vi "U3 Firmware Counter with Debounce.vi"() -> ()   [LabVIEW 2021]
panel:
  in  "Rising Edges":bool
  in  "Debounce Period Values":u8[](array[numeric])=[50, 50]
  out "Counter Reads":u32[](array[numeric])
  in  "Timer/Counter Pin Offset":u8=4
  in  "Reset Counters":bool
  in  "Iteration Inverval (ms)":u32=200
  out "Timer Value Reads":u32[](array[numeric])
  out "Iteration":i32=10
  in  "error in":errorcluster
  in  "Address":string="1"
  in  "FirstFound":bool=TRUE
  in  "stop":bool
  out "error out":errorcluster
  out "Error Message":string="No Error"
  # "Enables both firmware counters (timers) with debounce (mode 6) and both hardware counters, then reads\nall at the specified interval.  Timers will be assigned to pins starting with FIO0 plus pin offset, and the\nhardware counters will get the next two pins after the timers.\n\nThe \"Debounce Period Value\" species how many 16 ms increments in the debounce period.  With a value\nof 5, the debounce period is 80 ms.\n\nTest by connect a wire to GND, and then tapping it in the various input terminals.  The hardware counters will\nrecord many counts for each tap, but with the proper debounce period the firmware counters will only record one\ncount per tap."
  # "Firmware Counter 0"
  # "Firmware Counter 1"
  # "Counter 0"
  # "Counter 1"
  # "Firmware Counter 0"
  # "Firmware Counter 1"
  # "This VI passes a timer\nbase clock constant that\nis valid for hardware V1.21.\nFor hardware V1.20 change\nLJ_tc48MHZ to LJ_tc24MHZ."
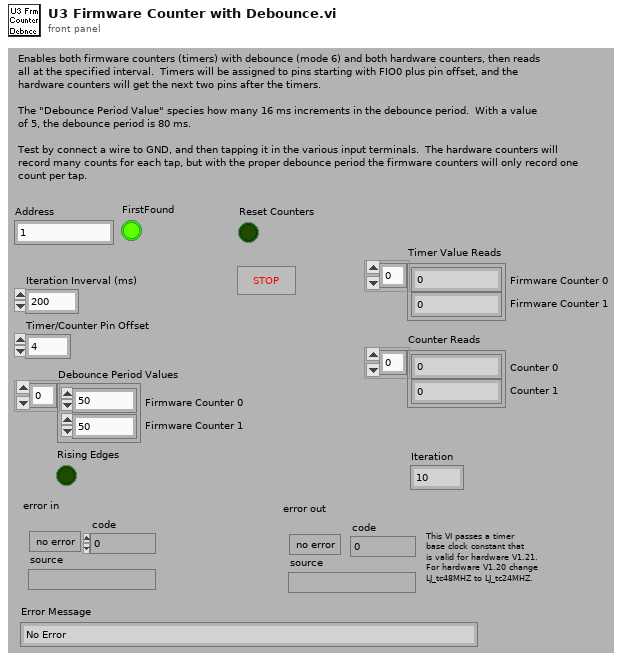
[diagram p1: front panel]
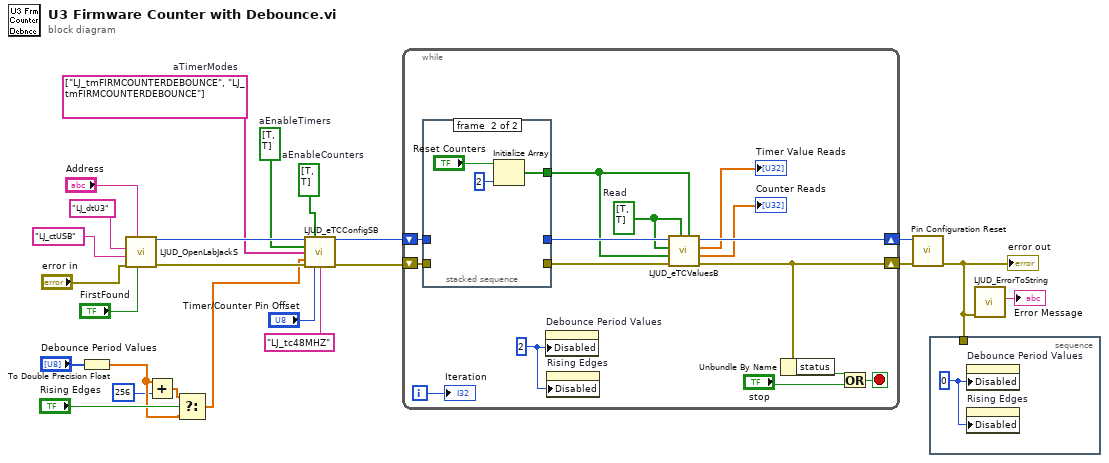
[diagram p0: block diagram]
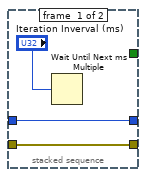
[diagram p2: hidden frame]
diagram:
  w11 = string[] ["LJ_tmFIRMCOUNTERDEBOUNCE", "LJ_tmFIRMCOUNTERDEBOUNCE"]  # aTimerModes
  w12 = bool[] [TRUE, TRUE]  # aEnableTimers
  w13 = bool[] [TRUE, TRUE]  # aEnableCounters
  n1 = To Double Precision Float(number="Debounce Period Values") -> (double precision float=w4:dbl[])
  n2 = call "LJUD_OpenLabJackS.vi"("FirstFound"="FirstFound", "Address"="Address", "error in"="error in", "ConnectionType"="LJ_ctUSB", "DeviceType"="LJ_dtU3") -> ("error out"=w17:errorcluster, "Handle"=w18:i32)  [unwired: 4 in, 1 out]
  n3 = Add(x=w4, y=256) -> (x+y=w5:dbl[])
  n4 = Select(t=w5, s="Rising Edges", f=w4) -> (s? t:f=w2:dbl[])
  n5 = call "LJUD_eTCConfigSB.vi"("Handle In"=w18, "aEnableCounters"=w13, "aEnableTimers"=w12, "aTimerModes"=w11, "aTimerValues"=w2, "error in"=w17, "TCPinOffset"="Timer/Counter Pin Offset", "TimerClockBase"="LJ_tc48MHZ") -> ("Handle Out"=w14:i32, "error out"=w15:errorcluster)  [unwired: 6 in]
  n6 = while {
    shift-left: w15 -> [w38]
    shift-right: [w32] -> w9
    shift-left: w14 -> [w39]
    shift-right: [w31] -> w10
    i -> [w34]
    stop <- w37 stop-if-true
    w25 = u8 2 ("Disabled")
    w28 = bool[] [TRUE, TRUE]  # Read
    n7 = stacked-sequence {
      tunnel: [w42 _] -> w30
      tunnel: [w41 _] -> w33
      tunnel: w39 -> [w42 _]
      tunnel: w38 -> [w41 _]
      tunnel: [_ w43] -> w29
      frame #0 {
        n8 = Wait Until Next ms Multiple(millisecond multiple="Iteration Inverval (ms)") -> ()  [unwired: 1 out]
      }
      frame #1 {
        n9 = Initialize Array("Reset Counters", 2 ("Dimension Size")) -> (w43:bool[])
      }
    }
    n10 = property on="Debounce Period Values" class="Arr (strict)"("Disabled"=w25) -> ()  [unwired: 2 in, 2 out]
    n11 = property on="Rising Edges" class="Bool (strict)"("Disabled"=w25) -> ()  [unwired: 2 in, 2 out]
    n12 = call "LJUD_eTCValuesB.vi"("aResetCounters"=w29, "aReadCounters"=w28, "error in"=w33, "aUpdateResetTimers"=w29, "aReadTimers"=w28, "Handle In"=w30) -> ("error out"=w32:errorcluster, "aCounterValues"=→"Counter Reads":dbl[], "aTimerValues Read"=→"Timer Value Reads":dbl[], "Handle Out"=w31:i32)  [unwired: 2 in]
    n13 = Unbundle By Name(w32) -> ("status"=w36:bool)
    n14 = Or(x=w36, y="stop") -> (x .or. y?=w37:bool)
    "Iteration" <- w34
  }
  n15 = call "Pin Configuration Reset.vi"("error in"=w9, "Handle In"=w10) -> ("error out"=w1:errorcluster)  [unwired: 8 in, 1 out]
  "error out" <- w1
  n16 = stacked-sequence {
    tunnel: w1 -> [_]
    frame #0 {
      w46 = u8 0 ("Disabled")
      n17 = property on="Debounce Period Values" class="Arr (strict)"("Disabled"=w46) -> ()  [unwired: 2 in, 2 out]
      n18 = property on="Rising Edges" class="Bool (strict)"("Disabled"=w46) -> ()  [unwired: 2 in, 2 out]
    }
  }
  n19 = call "LJUD_ErrorToString.vi"("error in"=w1) -> ("String"=→"Error Message":string)  [unwired: 10 in]
